vi "Assign NaN for chosen axes.vi"(1 "New value":dbl=nan format="%.6f", 2 "Queried axes":string[](array[string]), 3 "Values":dbl[](array[numeric]) format="%.6f", 4 "Axes subset":string[](array[string])) -> (14 "New values":dbl[](array[numeric]) format="%.6f")   [LabVIEW 2020]
doc: "This VI returns \"NaN\" for the given axes subset."
panel:
  # "This vi returns NaN or a given value for the given axes subset."
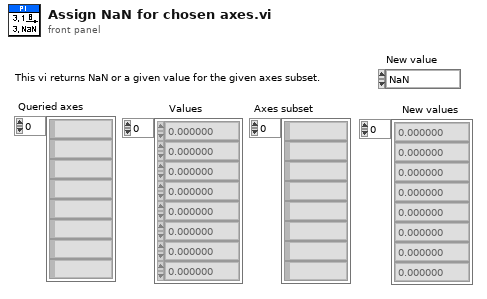
[diagram p1: front panel]
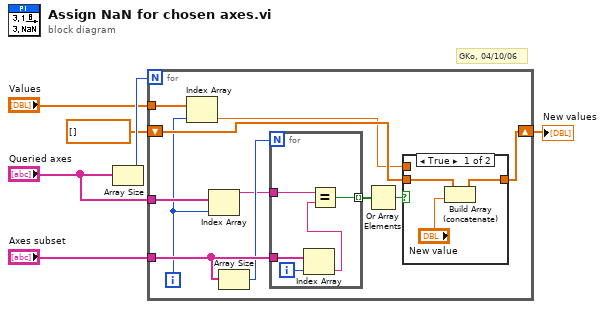
[diagram p0: block diagram]
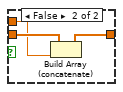
[diagram p2: hidden frame]
diagram:
  # "GKo, 04/10/06"
  n1 = Array Size(array="Queried axes") -> (size(s)=w6:i32)
  n2 = for {
    N: w6 -> [_]
    shift-right: [w12] -> w5
    shift-left: dbl[] [] -> [w11]
    tunnel: "Queried axes" -> [w17]
    tunnel: "Axes subset" -> [w16]
    tunnel: "Values" -> [w10]
    i -> [w9]
    n3 = Index Array(array=w10, index=w9) -> (element=w8:dbl)
    n4 = Index Array(array=w17, index=w9) -> (element=w7:string)
    n5 = Array Size(array=w16) -> (size(s)=w15:i32)
    n6 = for {
      N: w15 -> [_]
      tunnel: w7 -> [w24]
      tunnel: w16 -> [w28]
      tunnel: [w25] -> w14 mode=indexing
      i -> [w27]
      n7 = Index Array(array=w28, index=w27) -> (element=w26:string)
      n8 = Equal?(x=w24, y=w26) -> (x = y?=w25:bool)
    }
    n9 = Or Array Elements(Boolean array=w14) -> (logical OR=w13:bool)
    n10 = case shown="True" w13 {
      tunnel: [w20 w23] -> w12
      tunnel: w11 -> [w19 w22]
      tunnel: w8 -> [_ w21]
      frame True {
        n11 = Build Array (concatenate)(w19, "New value") -> (w20:dbl[])
      }
      frame False {
        n12 = Build Array (concatenate)(w22, w21) -> (w23:dbl[])
      }
    }
  }
  "New values" <- w5
